vi "test_ccd_trigger.vi"(8 "error in":errorcluster, 11 "CCD in":refnum<class "CCD.lvclass">) -> (0 "error out":errorcluster, 3 "CCD out":refnum<class "CCD.lvclass">)   [LabVIEW 2020, in "horiba.test.lvlib"]
uses:
  horiba.test.lvlib
  Classes/CCD/CCD.lvclass
  15e7fe39-3d4f-4ccc-ae5c-22e5f2c5c50b.vi
  ea63f925-e641-4c0a-a139-6263cd42ee73.vi
  Classes/CCD/TriggerIn.ctl
  0d1025e9-6526-4eb0-922b-3647fa86469f.vi
  0aa40d3a-c8ef-4f49-9493-ed4ba0189c53.vi
  <vilib>/addons/_JKI Toolkits/Caraya/classes/Assert/Assert Equal Value_Variant.vi
panel:
  # "Connector Pane"
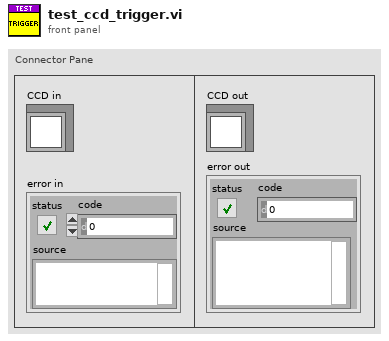
[diagram p1: front panel]
types:
  T1 = typedef "horiba.lvlib/CCD.lvclass/TriggerIn.ctl" = cluster{"address":i32, "event":i32, "signalType":i32}
  T2 = typedef "horiba.lvlib/CCD.lvclass/SignalOut.ctl" = cluster{"address":i32, "event":i32, "signalType":i32}
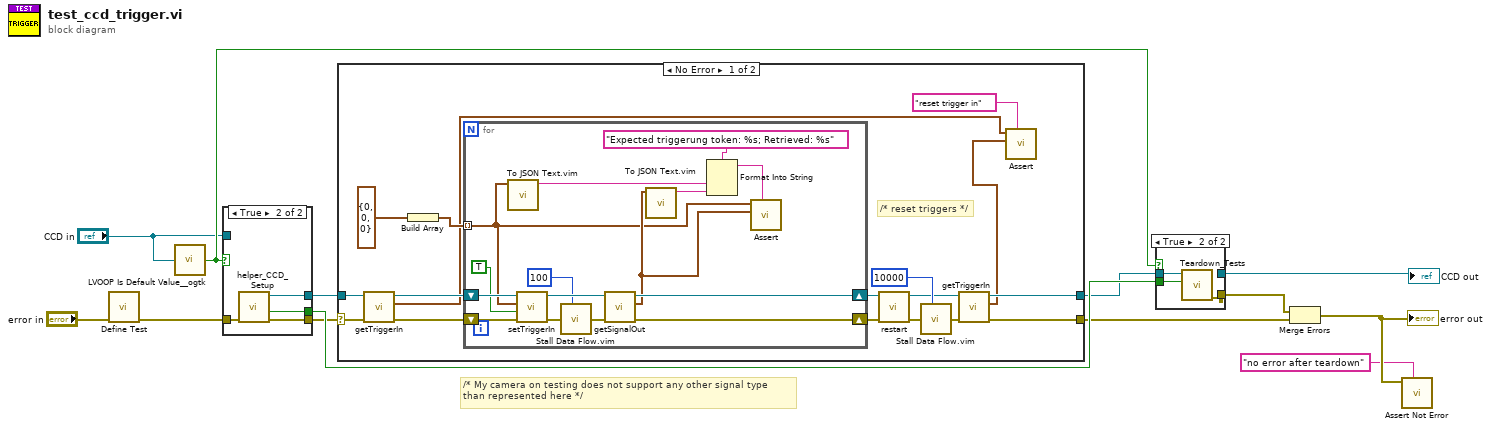
[diagram p0: block diagram]
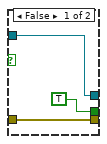
[diagram p3: hidden frame]
diagram:
  # "/* My camera on testing does not support any other signal type\nthan represented here */"
  n1 = call <vilib>:"Define Test.vi"("error in (no error)"="error in") -> ("error out"=w8:errorcluster)  [unwired: 9 in, 1 out]
  n2 = call <userlib>:"LVOOP Is Default Value__ogtk.vi"("Object"="CCD in") -> ("Is Default Value?"=w9:bool)
  n3 = case shown="True" w9 {
    tunnel: w8 -> [w15 w20]
    tunnel: [w15 w19] -> w4
    tunnel: [w16 w18] -> w6
    tunnel: [TRUE ("Module Was Already Running?") w17] -> w10
    tunnel: "CCD in" -> [w16 _]
    frame False {
    }
    frame True {
      n4 = call "helper_CCD_Setup.vi"("error in"=w20) -> ("error out"=w19:errorcluster, "Module Was Already Running?"=w17:bool, "CCD out"=w18:refnum<class "CCD.lvclass">)  [unwired: 7 in, 1 out]
    }
  }
  n5 = case shown="No Error" w4 {
    selector: w4 -> [w37 w53]
    tunnel: [w24 w54] -> w5
    tunnel: w6 -> [w36 w54]
    tunnel: [w26 w53] -> w3
    frame No Error {
      # "/* reset triggers */"
      n6 = call "getTriggerIn.vi"("error in (no error)"=w37, "CCD in"=w36) -> ("error out"=w34:errorcluster, "Trigger IN"=w22:T1, "CCD out"=w35:refnum<class "CCD.lvclass">)  [unwired: 7 in]
      n7 = Build Array(T1 {"address"=0, "event"=0, "signalType"=0} ("Trigger IN")) -> (w32:T1[])
      n8 = for {
        shift-right: [w49] -> w29
        shift-left: w35 -> [w50]
        shift-right: [w47] -> w33
        shift-left: w34 -> [w48]
        tunnel: w32 -> [w39] mode=indexing
        n9 = call "To JSON Text.vim"("Anything"=w39) -> ("<JSON>"=w42:string)  [unwired: 9 in, 1 out]
        n10 = call "setTriggerIn.vi"("error in (no error)"=w48, "enable"=TRUE, "Trigger IN"=w39, "CCD in"=w50) -> ("error out"=w52:errorcluster, "CCD out"=w51:refnum<class "CCD.lvclass">)  [unwired: 4 in, 2 out]
        n11 = call "Stall Data Flow.vim"("value in"=w52, "milliseconds to wait"=u32 100) -> ("value out"=w44:errorcluster)  [unwired: 1 out]
        n12 = call "getSignalOut.vi"("error in (no error)"=w44, "CCD in"=w51) -> ("error out"=w47:errorcluster, "Signal out"=w40:T2, "CCD out"=w49:refnum<class "CCD.lvclass">)  [unwired: 7 in]
        n13 = call "To JSON Text.vim"("Anything"=w40) -> ("<JSON>"=w41:string)  [unwired: 9 in, 1 out]
        n14 = Format Into String(format string="Expected triggerung token: %s; Retrieved: %s", w42, w41) -> (resulting string=w46:string)  [unwired: 2 in, 1 out]
        n15 = call-poly <vilib>:"Assert.vi"("Label"=w46, "Y"=w40, "X"=w39) -> ()  [unwired: 7 in, 2 out]
      }
      n16 = call "restart.vi"("error in (no error)"=w33, "CCD in"=w29) -> ("error out"=w30:errorcluster, "CCD out"=w25:refnum<class "CCD.lvclass">)  [unwired: 6 in, 2 out]
      n17 = call "Stall Data Flow.vim"("value in"=w30, "milliseconds to wait"=u32 10000) -> ("value out"=w28:errorcluster)  [unwired: 1 out]
      n18 = call "getTriggerIn.vi"("error in (no error)"=w28, "CCD in"=w25) -> ("error out"=w26:errorcluster, "Trigger IN"=w23:T1, "CCD out"=w24:refnum<class "CCD.lvclass">)  [unwired: 7 in]
      n19 = call-poly <vilib>:"Assert.vi"("Label"="reset trigger in", "Y"=w23, "X"=w22) -> ()  [unwired: 7 in, 2 out]
    }
    frame Error {
    }
  }
  n20 = case shown="True" w9 {
    tunnel: w5 -> [w55 w58]
    tunnel: [_ w57] -> w7
    tunnel: w10 -> [_ w56]
    tunnel: [w55 _] -> w1
    frame False {
    }
    frame True {
      n21 = call "Teardown_Tests.vi"("Module Was Already Running?"=w56, "horiba.lvlib:GenericDevice"=w58) -> ("error out"=w57:errorcluster)  [unwired: 8 in, 1 out]
    }
  }
  "CCD out" <- w1
  n22 = Merge Errors(w7, w3) -> (w12:errorcluster)
  "error out" <- w12
  n23 = call <vilib>:"Assert Not Error.vi"("Label"="no error after teardown", "Not Error?"=w12) -> ()  [unwired: 8 in, 2 out]
